vi "状态读取.vi"   [LabVIEW 2020]
uses:
  Global_Variable/Global.vi
types:
  T1 = cluster{"相机结果":dbl, "1":sgl, "工装移载位移":sgl, "1":sgl, "电缸位移":sgl, "345":sgl, "66":sgl, "一点":sgl, "拉压力":sgl, "发的":sgl}
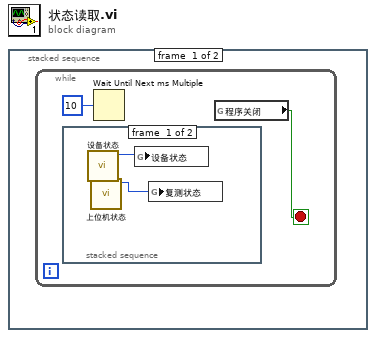
[diagram p0: block diagram]
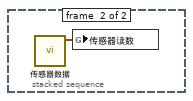
[diagram p2: hidden frame]
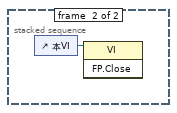
[diagram p3: hidden frame]
diagram:
  n1 = stacked-sequence {
    frame #0 {
      n2 = while {
        stop <- w1 stop-if-true
        n3 = stacked-sequence {
          frame #0 {
            n4 = call "设备状态.vi"() -> ("Status_Read"=w4:i16)  [unwired: 11 in]
            n5 = call "上位机状态.vi"() -> ("Status_Read"=w3:i16)  [unwired: 11 in]
            n6 = global write "Global.vi" "设备状态"(w4) -> ()
            n7 = global write "Global.vi" "复测状态"(w3) -> ()
          }
          frame #1 {
            n8 = call "传感器数据.vi"() -> ("传感器读数"=w5:T1)  [unwired: 11 in]
            n9 = global write "Global.vi" "传感器读数"(w5) -> ()
          }
        }
        n10 = Wait Until Next ms Multiple(millisecond multiple=u32 10 ("毫秒倍数")) -> ()  [unwired: 1 out]
        n11 = global read "Global.vi" "程序关闭"() -> (w1:bool)
      }
    }
    frame #1 {
      n12 = control-ref of="本VI"() -> (w6:refnum<vi>)
      n13 = invoke class="VI" method="FP.Close"(reference=w6) -> ()  [unwired: 2 in, 3 out]
    }
  }
